vi "Header Footer Add Cell.vi"(0 "PdfP Table":refnum<k24>, 1 "Header or Footer":T1, 5 "Page #":i32, 7 "Total page #":i32, 9 "Header Footer Cluster with references":T2={"Start page"=1, "Type"=enum."Select", "Alignment"=enum."Center", "Vertical Alignement"=enum."MIDDLE", "Page #"={"Text 1"="", "Text 2"="", "Text 3"=""}, "Text"=refnum, "Scaled Img"=refnum, "PdfPCell"=refnum, "PdfPTable"=refnum, "Font Cluster"={"Name"="", "Size"=-1.0, "Color"=0, "Style"={"Bold"=FALSE, "Italic"=FALSE, "Underline"=FALSE, "Strikeout"=FALSE}}, "Font "=refnum, "Img (%)"=100.0, "Line"={"Line"=enum."Horizontal line", "Thickness (points)"=0.75, "Colour"=7171459}}, 11 "error in (no error)":errorcluster) -> (4 "PdfP Table duplicate":refnum<k24>, 15 "error out":errorcluster)   [LabVIEW 2012]
doc: "Version 1.0\nDeveloped by Jean-Marc Simard\nCopyright © 2010, Exaprom Inc.\nAll rights reserved.\nLicense: BSD\n\nWith iTextSharp 4.1.6 (http://itextsharp.sourceforge.net)\nunder Mozilla Public License Version 1.1\n(http://www.mozilla.org/MPL/MPL-1.1.html)"
uses:
  C:/Users/MaxCorp/Documents/TopPerm - Base/DLL/itextsharp.dll
  DLL/itextsharp.dll
  Controls/Header Footer Cluster with references.ctl
  Controls/Header Footer Type.ctl
  Controls/Header footer horiz alignment.ctl
  Controls/Cell Vertical alignment.ctl
  Controls/Page number.ctl
  Controls/Font cluster.ctl
  Controls/Font size.ctl
  Controls/Font color.ctl
  Controls/Header Footer Line.ctl
  Controls/Header or Footer.ctl
panel:
  # "X"
  # "Y"
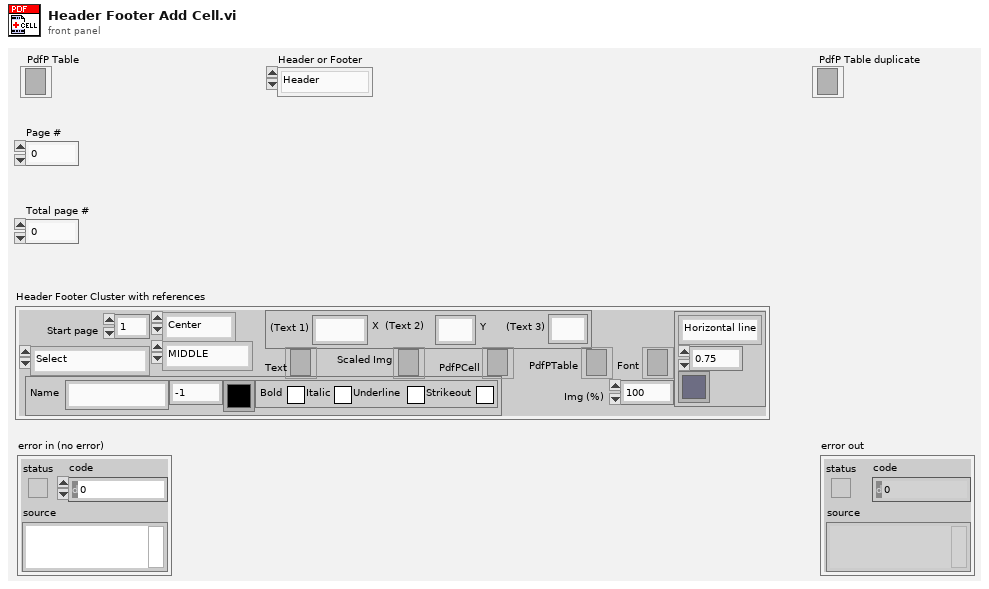
[diagram p1: front panel]
types:
  T1 = typedef "Header or Footer.ctl" = enum16{"Header", "Footer"}
  T2 = typedef "Header Footer Cluster with references.ctl" = cluster{"Start page":i32, "Type":T3, "Alignment":T4, "Vertical Alignement":T5, "Page #":T6, "Text":refnum<k24>, "Scaled Img":refnum<k24>, "PdfPCell":refnum<k24>, "PdfPTable":refnum<k24>, "Font Cluster":T7, "Font ":refnum<k24>, "Img (%)":sgl, "Line":cluster{"Line":T10, "Thickness (points)":sgl, "Colour":T9}}
  T3 = typedef "Header Footer Type.ctl" = enum16{"Select", "Text", "Text + hyperlink", "Page number", "Image", "Image + hyperlink"}
  T4 = typedef "Header footer horiz alignment.ctl" = enum16{"Left", "Center", "Right"}
  T5 = typedef "Cell Vertical alignment.ctl" = enum16{"TOP", "MIDDLE", "BOTTOM"}
  T6 = typedef "Page number.ctl" = cluster{"Text 1":string, "Text 2":string, "Text 3":string}
  T7 = typedef "Font cluster.ctl" = cluster{"Name":string, "Size":T8, "Color":T9, "Style":cluster{"Bold":bool, "Italic":bool, "Underline":bool, "Strikeout":bool}}
  T8 = typedef "Font size.ctl" = sgl
  T9 = typedef "Font color.ctl" = u32
  T10 = typedef "Header Footer Line.ctl" = enum16{"No line", "Horizontal line"}
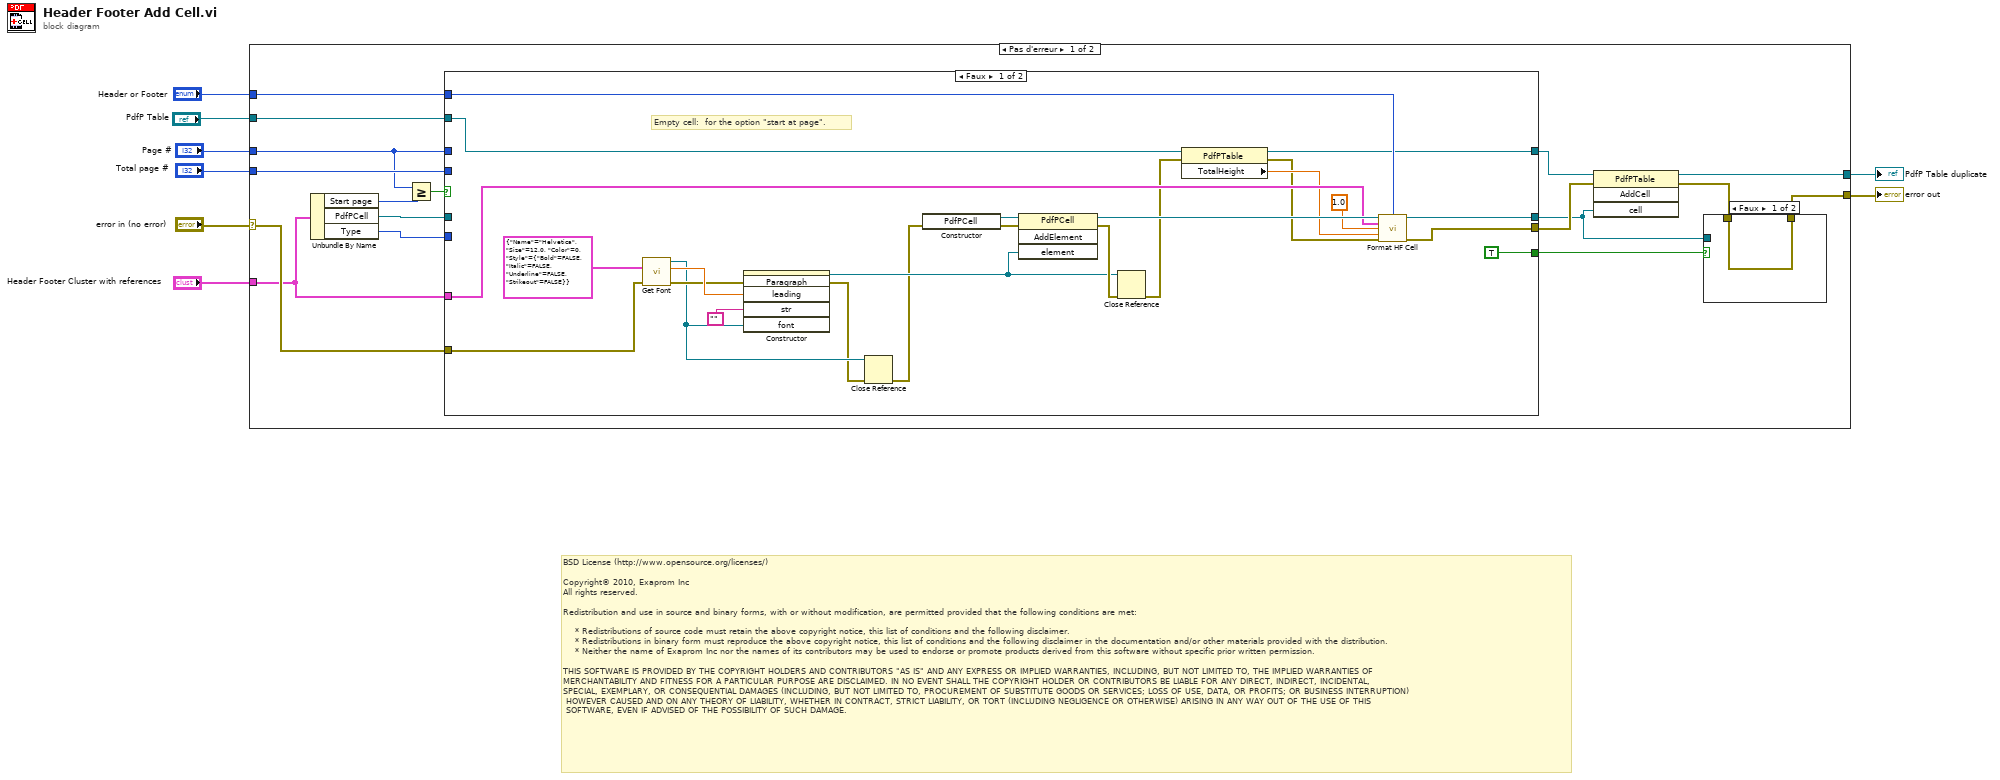
[diagram p0: block diagram]
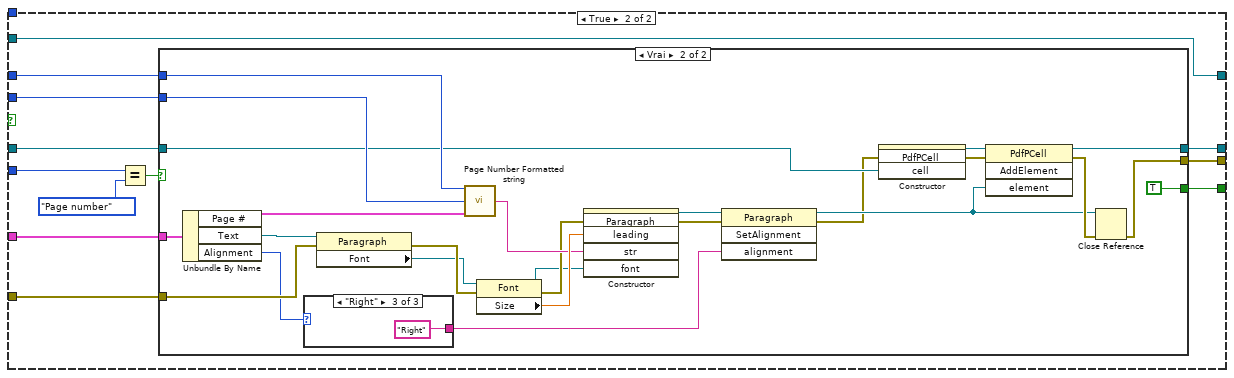
[diagram p2: hidden frame]
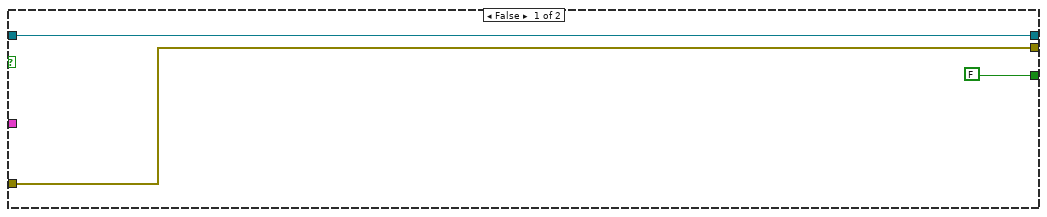
[diagram p3: hidden frame]
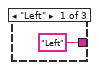
[diagram p4: hidden frame]
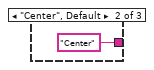
[diagram p5: hidden frame]
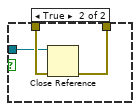
[diagram p6: hidden frame]
diagram:
  # "BSD License (http://www.opensource.org/licenses/)\n\nCopyright© 2010, Exaprom Inc\nAll rights reserved.\n\nRedistribution and use in source and binary forms, with or without modification, are permitted provided that the following conditions are met:\n\n    * Redistributions of source code must retain the above copyright notice, this list of conditions and the following disclaimer.\n    * Redistributions in binary form must reproduce the above copyright notice, this list of conditions and the following disclaimer in the documentation and/or other materials provided with the distribution.\n    * Neither the name of Exaprom Inc nor the names of its contributors may be used to endorse or promote products derived from this software without specific prior written permission.\n\nTHIS SOFTWARE IS PROVIDED BY THE COPYRIGHT HOLDERS AND CONTRIBUTORS \"AS IS\" AND ANY EXPRESS OR IMPLIED WARRANTIES, INCLUDING, BUT NOT LIMITED TO, THE IMPLIED WARRANTIES OF \nMERCHANTABILITY AND FITNESS FOR A PARTICULAR PURPOSE ARE DISCLAIMED. IN NO EVENT SHALL THE COPYRIGHT HOLDER OR CONTRIBUTORS BE LIABLE FOR ANY DIRECT, INDIRECT, INCIDENTAL,\nSPECIAL, EXEMPLARY, OR CONSEQUENTIAL DAMAGES (INCLUDING, BUT NOT LIMITED TO, PROCUREMENT OF SUBSTITUTE GOODS OR SERVICES; LOSS OF USE, DATA, OR PROFITS; OR BUSINESS INTERRUPTION)\n HOWEVER CAUSED AND ON ANY THEORY OF LIABILITY, WHETHER IN CONTRACT, STRICT LIABILITY, OR TORT (INCLUDING NEGLIGENCE OR OTHERWISE) ARISING IN ANY WAY OUT OF THE USE OF THIS\n SOFTWARE, EVEN IF ADVISED OF THE POSSIBILITY OF SUCH DAMAGE."
  n1 = case shown="Pas d'erreur" "error in (no error)" {
    selector: "error in (no error)" -> [w19 w98]
    tunnel: "Header Footer Cluster with references" -> [w18 _]
    tunnel: "Page #" -> [w13 _]
    tunnel: "Total page #" -> [w20 _]
    tunnel: [w22 w98] -> w5
    tunnel: [w24 w97] -> w2
    tunnel: "PdfP Table" -> [w10 w97]
    tunnel: "Header or Footer" -> [w11 _]
    frame No Error {
      n2 = Unbundle By Name(w18) -> ("Start page"=w14:i32, "PdfPCell"=w15:refnum<k24>, "Type"=w16:T3)
      n3 = Greater Or Equal?(x=w13, y=w14) -> (x >= y?=w12:bool)
      n4 = case shown="Faux" w12 {
        tunnel: [w34 w61] -> w25
        tunnel: [w35 w60] -> w21
        tunnel: w20 -> [_ w59]
        tunnel: w19 -> [w41 w58]
        tunnel: w18 -> [w32 w57]
        tunnel: [TRUE w56] -> w17
        tunnel: w16 -> [_ w54]
        tunnel: w15 -> [_ w52]
        tunnel: w13 -> [_ w51]
        tunnel: w11 -> [w33 _]
        tunnel: w10 -> [w30 w50]
        tunnel: [w28 w50] -> w9
        frame False {
          # "Empty cell:  for the option \"start at page\"."
          n5 = call "Get Font.vi"("error in (no error)"=w41, "Font IN"=T7 {"Name"="Helvetica", "Size"=12.0, "Color"=0, "Style"={"Bold"=FALSE, "Italic"=FALSE, "Underline"=FALSE, "Strikeout"=FALSE}}) -> ("error out"=w40:errorcluster, "Font Size"=w44:T8, "Font"=w39:refnum<k24>)  [unwired: 1 in, 6 out]
          n6 = constructor class="Paragraph"(error in=w40, "leading"=w44, "str"="", "font"=w39) -> (reference out=w45:refnum<k24>, error out=w38:errorcluster)  [unwired: 2 in, 4 out]
          n7 = Close Reference(reference=w39, error in (no error)=w38) -> (error out=w37:errorcluster)
          n8 = constructor class="PdfPCell"(error in=w37) -> (reference out=w47:refnum<k24>, error out=w46:errorcluster)  [unwired: 2 in, 1 out]
          n9 = invoke class="PdfPCell" method="AddElement"(reference=w47, error in=w46, "element"=w45) -> (reference out=w36:refnum<k24>, error out=w48:errorcluster)  [unwired: 1 in, 2 out]
          n10 = Close Reference(reference=w45, error in (no error)=w48) -> (error out=w27:errorcluster)
          n11 = property class="PdfPTable"(reference=w30, error in=w27) -> (reference out=w28:refnum<k24>, error out=w26:errorcluster, "TotalHeight"=w29:sgl)
          n12 = call "Format HF Cell.vi"("PdfP Cell"=w36, "Header or Footer"=w33, "Header Footer Cluster with references"=w32, "Padding (points)"=sgl 1.0 ("FixedHeight (points)"), "FixedHeight (points)"=w29, "error in (no error)"=w26) -> ("PdfP Cell duplicate"=w35:refnum<k24>, "error out"=w34:errorcluster)  [unwired: 8 out]
        }
        frame True {
          n13 = Equal?(x=w54, y=Header_Footer_Type."Page number" ("x")) -> (x = y?=w55:bool)
          n14 = case shown="Vrai" w55 {
            tunnel: w52 -> [w64 w70]
            tunnel: [w64 w89] -> w60
            tunnel: w57 -> [_ w88]
            tunnel: w59 -> [_ w86]
            tunnel: w51 -> [_ w85]
            tunnel: w58 -> [w63 w78]
            tunnel: [w63 w68] -> w61
            tunnel: [FALSE TRUE] -> w56
            frame False {
            }
            frame True {
              n15 = Unbundle By Name(w88) -> ("Page #"=w87:T6, "Text"=w83:refnum<k24>, "Alignment"=w77:T4)
              n16 = case shown="\"Right\"" w77 {
                tunnel: ["Left" "Center" "Right"] -> w72
                frame "Left" {
                }
                frame "Center", Default {
                }
                frame "Right" {
                }
              }
              n17 = property class="Paragraph"(reference=w83, error in=w78) -> (error out=w82:errorcluster, "Font"=w80:refnum<k24>)  [unwired: 1 out]
              n18 = call "Page Number Formatted string.vi"("Page #"=w85, "Total page #"=w86, "Page # cluster"=w87) -> ("Page string"=w79:string)  [unwired: 12 out]
              n19 = property class="Font"(reference=w80, error in=w82) -> (reference out=w73:refnum<k24>, error out=w74:errorcluster, "Size"=w81:sgl)
              n20 = constructor class="Paragraph"(error in=w74, "leading"=w81, "str"=w79, "font"=w73) -> (reference out=w76:refnum<k24>, error out=w75:errorcluster)  [unwired: 2 in, 4 out]
              n21 = invoke class="Paragraph" method="SetAlignment"(reference=w76, error in=w75, "alignment"=w72) -> (reference out=w71:refnum<k24>, error out=w65:errorcluster)  [unwired: 1 in, 2 out]
              n22 = constructor class="PdfPCell"(error in=w65, "cell"=w70) -> (reference out=w69:refnum<k24>, error out=w66:errorcluster)  [unwired: 2 in, 2 out]
              n23 = invoke class="PdfPCell" method="AddElement"(reference=w69, error in=w66, "element"=w71) -> (reference out=w89:refnum<k24>, error out=w84:errorcluster)  [unwired: 1 in, 2 out]
              n24 = Close Reference(reference=w71, error in (no error)=w84) -> (error out=w68:errorcluster)
            }
          }
        }
      }
      n25 = invoke class="PdfPTable" method="AddCell"(reference=w9, error in=w25, "cell"=w21) -> (reference out=w24:refnum<k24>, error out=w23:errorcluster)  [unwired: 1 in, 2 out]
      n26 = case shown="Faux" w17 {
        tunnel: w23 -> [w93 w96]
        tunnel: [w93 w95] -> w22
        tunnel: w21 -> [_ w94]
        frame False {
        }
        frame True {
          n27 = Close Reference(reference=w94, error in (no error)=w96) -> (error out=w95:errorcluster)
        }
      }
    }
    frame Error {
    }
  }
  "error out" <- w5
  "PdfP Table duplicate" <- w2
